vi "CallVSGateway.vi"   [LabVIEW 2011]
panel:
  # "This EXE calls the VS gateway silently"
  # "SilentVeriStand.EXE"
types:
  T1 = enum32{"Invalid", "Standard", "Closed", "Hidden", "Minimized", "Maximized"}
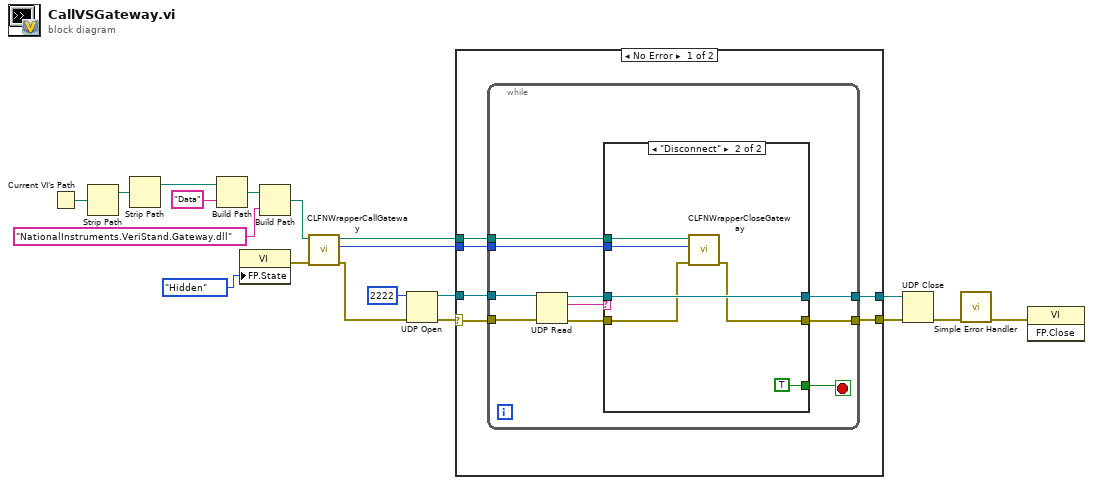
[diagram p0: block diagram]
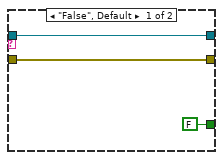
[diagram p2: hidden frame]
diagram:
  n1 = Current VI's Path() -> (path=w11:path)
  n2 = Strip Path(path=w11) -> (stripped path=w10:path)  [unwired: 1 out]
  n3 = Strip Path(path=w10) -> (stripped path=w9:path)  [unwired: 1 out]
  n4 = Build Path(base path=w9, name or relative path="Data") -> (appended path=w7:path)
  n5 = property class="VI"("FP.State"=T1."Hidden" ("State")) -> (error out=w1:errorcluster)  [unwired: 2 in, 1 out]
  n6 = Build Path(base path=w7, name or relative path="NationalInstruments.VeriStand.Gateway.dll") -> (appended path=w5:path)
  n7 = call "CLFNWrapperCallGateway.vi"("error in (no error)"=w1, "appended path"=w5) -> ("error out"=w2:errorcluster, "ref"=w19:i32, "path out"=w4:path)  [unwired: 7 in]
  n8 = UDP Open(8:w2, 11:u16 2222 ("port")) -> (port=w18:refnum<k16>, 0:w14:errorcluster)  [unwired: 3 in, 1 out]
  n9 = case shown="No Error" w14 {
    selector: w14 -> [w21 w46]
    tunnel: w19 -> [w25 _]
    tunnel: w18 -> [w24 w45]
    tunnel: [w23 w46] -> w16
    tunnel: [w22 w45] -> w15
    tunnel: w4 -> [w20 _]
    frame No Error {
      n10 = while {
        tunnel: w25 -> [w32]
        tunnel: w24 -> [w35]
        tunnel: w21 -> [w34]
        tunnel: [w29] -> w23
        tunnel: [w27] -> w22
        tunnel: w20 -> [w26]
        stop <- w31 stop-if-true
        n11 = UDP Read(connection ID=w35, 8:w34) -> (data out=w33:string, error out=w30:errorcluster, 3:w28:refnum<k16>)  [unwired: 2 in, 2 out]
        n12 = case shown="\"Disconnect\"" w33 {
          tunnel: w32 -> [_ w44]
          tunnel: [FALSE TRUE] -> w31
          tunnel: w30 -> [w37 w41]
          tunnel: [w37 w40] -> w29
          tunnel: w28 -> [w36 w42]
          tunnel: [w36 w42] -> w27
          tunnel: w26 -> [_ w39]
          frame "False", Default {
          }
          frame "Disconnect" {
            n13 = call "CLFNWrapperCloseGateway.vi"("error in (no error)"=w41, "ref"=w44, "path out"=w39) -> ("error out"=w40:errorcluster)  [unwired: 8 in]
          }
        }
      }
    }
    frame Error {
    }
  }
  n14 = UDP Close(connection ID=w15, 8:w16) -> (error out=w13:errorcluster)  [unwired: 1 out]
  n15 = call <vilib>:"Simple Error Handler.vi"("error in (no error)"=w13) -> ("error out"=w12:errorcluster)  [unwired: 4 in, 4 out]
  n16 = invoke class="VI" method="FP.Close"(error in=w12) -> ()  [unwired: 2 in, 3 out]
